vi "Main.vi"(8 "error in (no error)":errorcluster, 11 "Stop notifier":refnum<notifier>) -> (0 "error out":errorcluster)   [LabVIEW 2017, in "WebRead.lvlib"]
doc: "Module main"
uses:
  WebRead.lvlib
  ctl/StateData.ctl
  ctl/MainStates.ctl
  ctl/JSONForm.ctl
  <vilib>/ErrorRing/Error Ring.xnode
  Error/Error.lvlib
panel:
  out "time stamp":timestamp
  out "USD":dbl format="%#_15g"
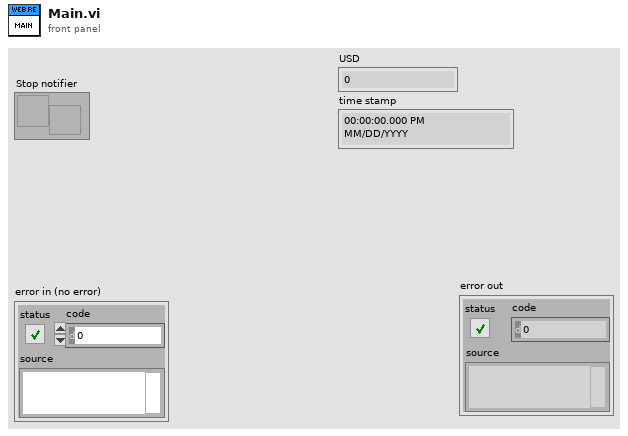
[diagram p1: front panel]
types:
  T1 = typedef "WebRead.lvlib/StateData.ctl" = cluster{"Blank":dbl}
  T2 = typedef "WebRead.lvlib/JSONForm.ctl" = cluster{"bpi":cluster{"USD":cluster{"rate":string}}, "time":cluster{"updatedISO":string}}
  T3 = typedef "WebRead.lvlib/MainStates.ctl" = enum16{"Timeout", "Error", "Exit", "Init", "ReadJSON", "ProcessJSON"}
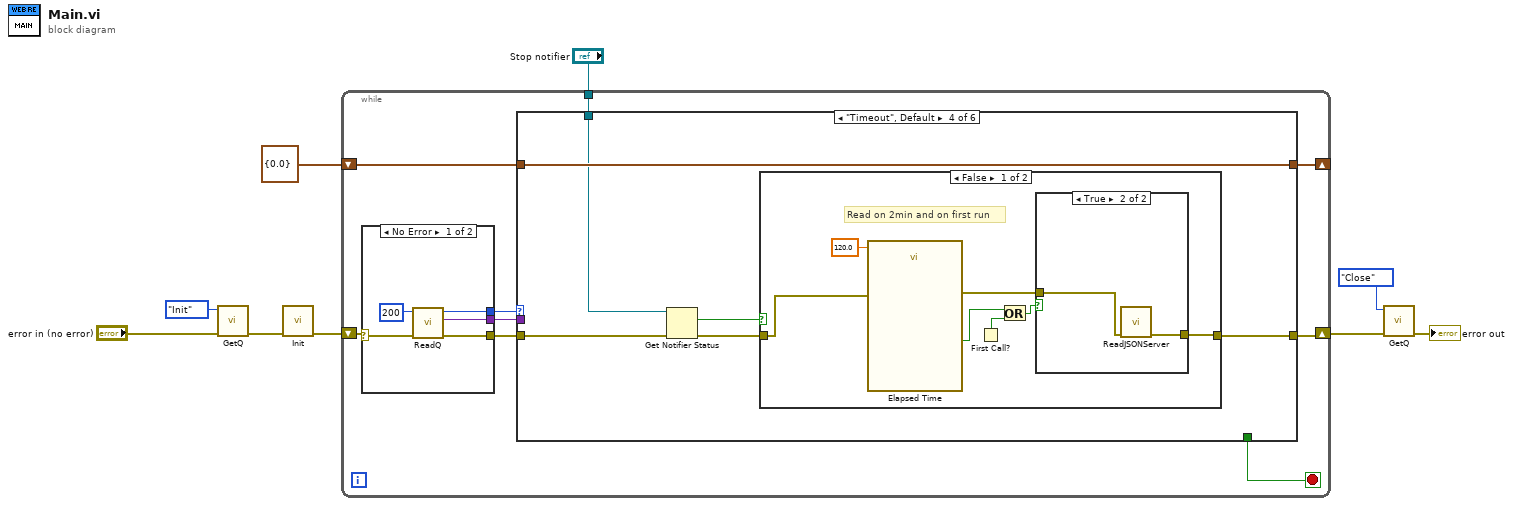
[diagram p0: block diagram]
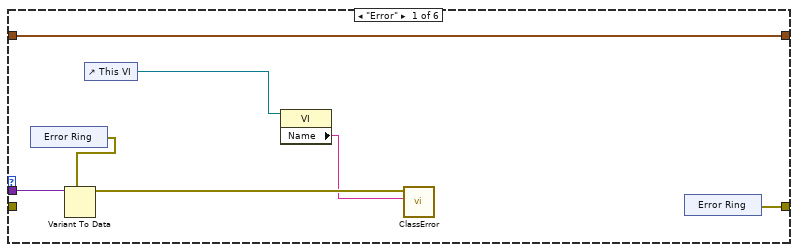
[diagram p2: hidden frame]
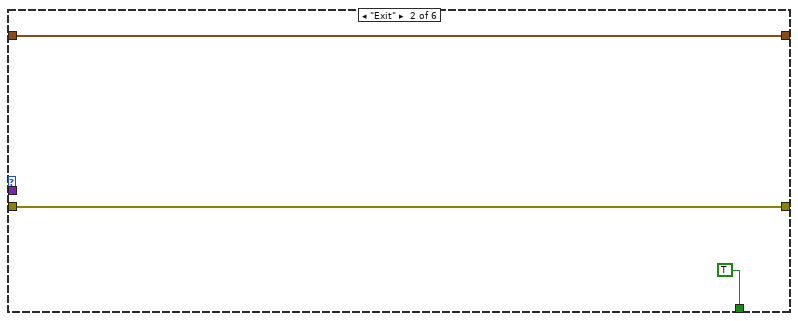
[diagram p3: hidden frame]
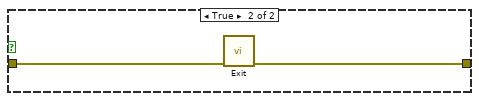
[diagram p6: hidden frame]
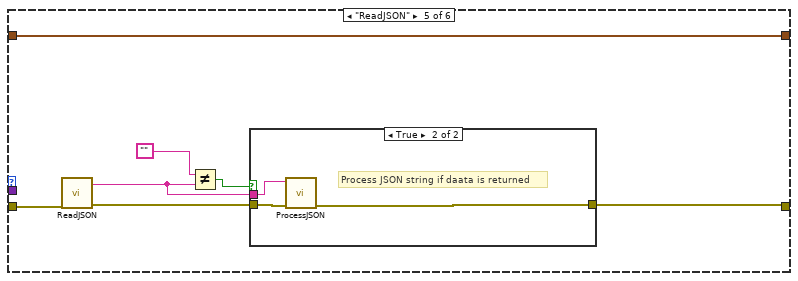
[diagram p7: hidden frame]
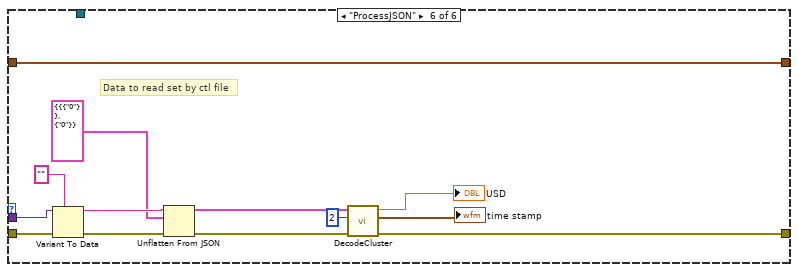
[diagram p9: hidden frame]
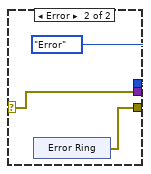
[diagram p10: hidden frame]
diagram:
  n1 = call "GetQ.vi"("error in (no error)"="error in (no error)", "Mode (Get)"=enum16{"Get", "Close", "Init"}."Init") -> ("error out"=w2:errorcluster)  [unwired: 8 in, 1 out]
  n2 = call "Init.vi"("error in (no error)"=w2) -> ("error out"=w1:errorcluster)  [unwired: 10 in]
  n3 = while {
    shift-right: [w14] -> w6
    shift-left: w1 -> [w18]
    shift-right: [w11] -> _
    shift-left: T1 {"Blank"=0.0} ("Cluster") -> [w12]
    tunnel: "Stop notifier" -> [w10]
    stop <- w13 stop-if-true
    n4 = case shown="No Error" w18 {
      selector: w18 -> [w79 w81]
      tunnel: [w78 MainStates."Error" ("State")] -> w17
      tunnel: [w77 w81] -> w16
      tunnel: [w76 w80] -> w15
      frame No Error {
        n5 = call "ReadQ.vi"("error in (no error)"=w79, "timeout in ms (200)"=200) -> ("error out"=w76:errorcluster, "Variant"=w77:variant, "State"=w78:T3)  [unwired: 7 in]
      }
      frame Error {
        n6 = xnode "Error Ring"() -> ("error out"=w80:errorcluster)
      }
    }
    n7 = case shown="\"Timeout\", Default" w17 {
      tunnel: w16 -> [w25 _ _ _ _ w72]
      tunnel: w15 -> [_ w30 w32 w37 w56 w73]
      tunnel: [w24 w30 w32 w34 w52 w62] -> w14
      tunnel: [_ TRUE _ _ _ _] -> w13
      tunnel: w12 -> [w22 w28 w31 w38 w57 w74]
      tunnel: [w22 w28 w31 w38 w57 w74] -> w11
      tunnel: w10 -> [_ _ _ w36 _ _]
      frame "Error" {
        n8 = xnode "Error Ring"() -> ("error out"=w23:errorcluster)
        n9 = Variant To Data(type=w23, Variant=w25) -> (data=w21:errorcluster)  [unwired: 1 in, 1 out]
        n10 = control-ref of="This VI"() -> (w20:refnum<vi>)
        n11 = property class="VI"(reference=w20) -> ("Name"=w19:string)  [unwired: 1 in, 2 out]
        n12 = call "ClassError.vi"("From"=w19, "error in"=w21) -> ()  [unwired: 9 in, 1 out]
        n13 = xnode "Error Ring"() -> ("error out"=w24:errorcluster)
      }
      frame "Exit" {
      }
      frame "Init" {
      }
      frame "Timeout", Default {
        n14 = Get Notifier Status(notifier=w36, error in (no error)=w37) -> (current notification=w35:bool, error out=w33:errorcluster)  [unwired: 3 out]
        n15 = case shown="False" w35 {
          tunnel: [w45 w49] -> w34
          tunnel: w33 -> [w39 w50]
          frame False {
            # "Read on 2min and on first run"
            n16 = call "Elapsed Time"("Time Target (s)"=120.0, "error in (no error)"=w39) -> ("Time has Elapsed"=w42:bool, "error out"=w44:errorcluster)  [unwired: 10 in, 6 out]
            n17 = First Call?() -> (First Call?: T/F=w41:bool)
            n18 = Or(x=w42, y=w41) -> (x .or. y?=w43:bool)
            n19 = case shown="True" w43 {
              tunnel: [w46 w48] -> w45
              tunnel: w44 -> [w46 w47]
              frame False {
                # "do nothing if time\nhas not passed"
              }
              frame True {
                n20 = call "ReadJSONServer.vi"("error in (no error)"=w47) -> ("error out"=w48:errorcluster)  [unwired: 10 in]
              }
            }
          }
          frame True {
            n21 = call "Exit.vi"("error in (no error)"=w50) -> ("error out"=w49:errorcluster)  [unwired: 10 in]
          }
        }
      }
      frame "ReadJSON" {
        n22 = call "ReadJSON.vi"("error in (no error)"=w56) -> ("error out"=w54:errorcluster, "JSON out"=w53:string)  [unwired: 9 in]
        n23 = Not Equal?(x="", y=w53) -> (x != y?=w51:bool)
        n24 = case shown="True" w51 {
          tunnel: w54 -> [w58 w61]
          tunnel: w53 -> [_ w60]
          tunnel: [w58 w59] -> w52
          frame False {
            # "no data"
          }
          frame True {
            # "Process JSON string if daata is returned"
            n25 = call "ProcessJSON.vi"("error in (no error)"=w61, "JASONdata"=w60) -> ("error out"=w59:errorcluster)  [unwired: 9 in]
          }
        }
      }
      frame "ProcessJSON" {
        # "Data to read set by ctl file"
        n26 = Variant To Data(error in=w73, type="" ("name"), Variant=w72) -> (data=w70:string, error out=w69:errorcluster)
        n27 = Unflatten From JSON(JSON string=w70, type and defaults=T2 {"bpi"={"USD"={"rate"="0"}}, "time"={"updatedISO"="0"}} ("value"), error in (no error)=w69) -> (value=w67:T2, error out=w63:errorcluster)  [unwired: 4 in]
        n28 = call "DecodeCluster.vi"("error in (no error)"=w63, "TimeZone"=2, "value"=w67) -> ("error out"=w62:errorcluster, "time stamp"=→"time stamp":timestamp, "USD"=→"USD":dbl)  [unwired: 6 in]
      }
    }
  }
  n29 = call "GetQ.vi"("error in (no error)"=w6, "Mode (Get)"=enum16{"Get", "Close", "Init"}."Close") -> ("error out"=→"error out":errorcluster)  [unwired: 8 in, 1 out]
